vi "NNScoreImage.vi"(0 "lookup path":path, 1 "Window Av Size":i8=3, 2 "psa":dbl format="%.2f", 3 "Intercept":dbl[][](array[numeric]) format="%.2f", 4 "MidBand":dbl[][](array[numeric]) format="%.2f") -> (6 "score":dbl[][](graph), 7 "Range Params":T1={"mb max"=-10.0, "mb min"=-60.0, "slope max"=4.0, "slope min"=-8.0, "int max"=5.0, "int min"=-85.0} {"int min" format="%.2f"; "int max" format="%.2f"; "slope min" format="%.2f"; "slope max" format="%.2f"; "mb min" format="%.2f"; "mb max" format="%.2f"}, 10 "Range Params in LUT":T1={"mb max"=-20.0, "mb min"=-70.0, "slope max"=8.0, "slope min"=-8.0, "int max"=5.0, "int min"=-85.0} {"int min" format="%.2f"; "int max" format="%.2f"; "slope min" format="%.2f"; "slope max" format="%.2f"; "mb min" format="%.2f"; "mb max" format="%.2f"})   [LabVIEW 2022 SP3]
uses:
  <vilib>/Utility/file.llb/Read Delimited Spreadsheet (DBL).vi
panel:
  out "min score":sgl
  out "max score":sgl
  in  "Look Up Dimension":i32=40
  out "Look up Table":dbl[][][](array[numeric]) format="%.6f"
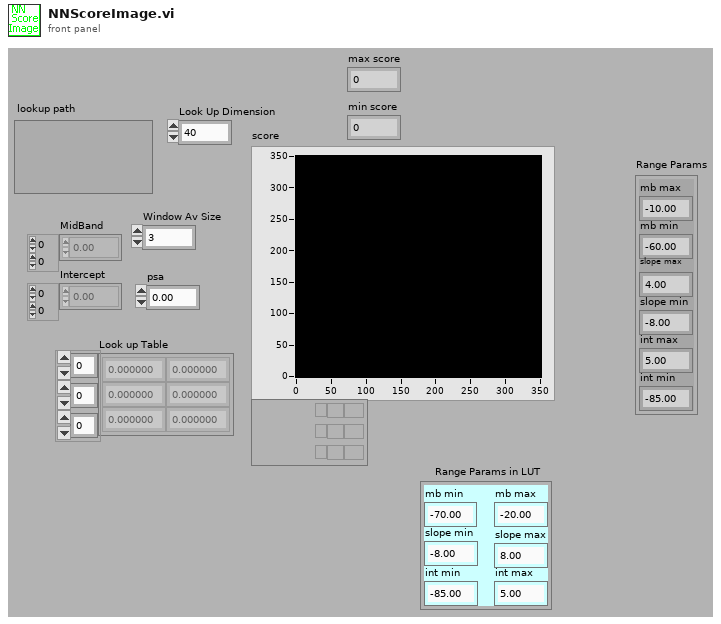
[diagram p1: front panel]
types:
  T1 = cluster{"mb max":dbl, "mb min":dbl, "slope max":dbl, "slope min":dbl, "int max":dbl, "int min":dbl}
  T2 = cluster{"[0]":dbl, "[1]":dbl, "[2]":dbl, "[3]":dbl, "[4]":dbl, "[5]":dbl, "[6]":dbl, "[7]":dbl}
  T3 = cluster{"[5]":dbl, "[4]":dbl, "[1]":dbl, "[0]":dbl, "[3]":dbl, "[2]":dbl}
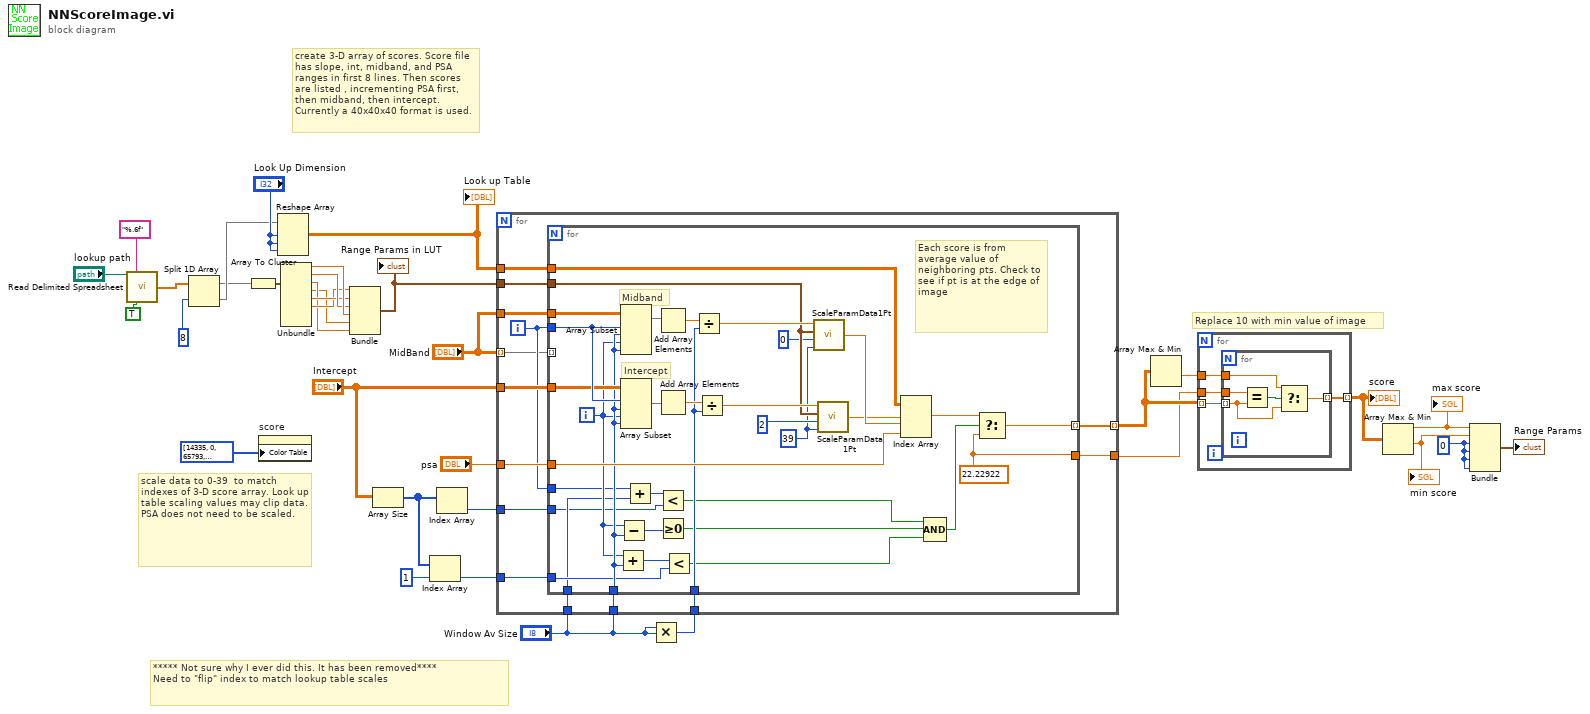
[diagram p0: block diagram]
diagram:
  w8 = 0
  # "***** Not sure why I ever did this. It has been removed****\nNeed to \"flip\" index to match lookup table scales"
  # "Replace 10 with min value of image"
  # "scale data to 0-39  to match indexes of 3-D score array. Look up table scaling values may clip data. PSA does not need to be scaled."
  # "create 3-D array of scores. Score file has slope, int, midband, and PSA ranges in first 8 lines. Then scores are listed , incrementing PSA first, then midband, then intercept.  Currently a 40x40x40 format is used."
  n1 = call-poly <vilib>:"Read Delimited Spreadsheet.vi"("file path (dialog if empty)"="lookup path", "format (%.3f)"="%.6f", "transpose? (F)"=TRUE) -> ("first row"=w7:dbl[])  [unwired: 7 in, 5 out]
  n2 = Split 1D Array(array=w7, index=8) -> (first subarray=w4:dbl[], second subarray=w5:dbl[])
  n3 = Array To Cluster(array=w4) -> (cluster=w32:T2)
  n4 = property on="score" class="IntGraph (strict)"("Color Table"=u32[] [14335, 0, 65793, 131586, 197379, 263172, 328965, 394758, 460551, 526344, 592137, 657930, 723723, 789516, 855309, 921102, 986895, 1052688, 1118481, 1184274, 1250067, 1315860, 1381653, 1447446, 1513239, 1579032, 1644825, 1710618, 1776411, 1842204, 1907997, 1973790, 2039583, 2105376, 2171169, 2236962, 2302755, 2368548, 2434341, 2500134, 2565927, 2631720, 2697513, 2763306, 2829099, 2894892, 2960685, 3026478, 3092271, 3158064, 3223857, 3289650, 3355443, 3421236, 3487029, 3552822, 3618615, 3684408, 3750201, 3815994, 3881787, 3947580, 4013373, 4079166, 4144959, 4210752, 4276545, 4342338, 4408131, 4473924, 4539717, 4605510, 4671303, 4737096, 4802889, 4868682, 4934475, 5000268, 5066061, 5131854, 5197647, 5263440, 5329233, 5395026, 5460819, 5526612, 5592405, 5658198, 5723991, 5789784, 5855577, 5921370, 5987163, 6052956, 6118749, 6184542, 6250335, 6316128, 6381921, 6447714, 6513507, 6579300, 6645093, 6710886, 6776679, 6842472, 6908265, 6974058, 7039851, 7105644, 7171437, 7237230, 7303023, 7368816, 7434609, 7500402, 7566195, 7631988, 7697781, 7763574, 7829367, 7895160, 7960953, 8026746, 8092539, 8158332, 8224125, 8289918, 8355711, 8421504, 8487297, 8553090, 8618883, 8684676, 8750469, 8816262, 8882055, 8947848, 9013641, 9079434, 9145227, 9211020, 9276813, 9342606, 9408399, 9474192, 9539985, 9605778, 9671571, 9737364, 9803157, 9868950, 9934743, 10000536, 10066329, 10132122, 10197915, 10263708, 10329501, 10395294, 10461087, 10526880, 10592673, 10658466, 10724259, 10790052, 10855845, 10921638, 10987431, 11053224, 11119017, 11184810, 11250603, 11316396, 11382189, 11447982, 11513775, 11579568, 11645361, 11711154, 11776947, 11842740, 11908533, 11974326, 12040119, 12105912, 12171705, 12237498, 12303291, 12369084, 12434877, 12500670, 12566463, 12632256, 12698049, 12763842, 12829635, 12895428, 12961221, 13027014, 13092807, 13158600, 13224393, 13290186, 13355979, 13421772, 13487565, 13553358, 13619151, 13684944, 13750737, 13816530, 13882323, 13948116, 14013909, 14079702, 14145495, 14211288, 14277081, 14342874, 14408667, 14474460, 14540253, 14606046, 14671839, 14737632, 14803425, 14869218, 14935011, 15000804, 15066597, 15132390, 15198183, 15263976, 15329769, 15395562, 15461355, 15527148, 15592941, 15658734, 15724527, 15790320, 15856113, 15921906, 15987699, 16053492, 16119285, 16185078, 16250871, 16316664, 16382457, 16448250, 16514043, 16579836, 16758546, 16711731]) -> ()  [unwired: 2 in, 2 out]
  n5 = Reshape Array(w5, "Look Up Dimension", "Look Up Dimension", "Look Up Dimension") -> (w10:dbl[][][])
  "Look up Table" <- w10
  n6 = Unbundle(w32) -> ("[0]"=w31:dbl, "[1]"=w30:dbl, "[2]"=w27:dbl, "[3]"=w26:dbl, "[4]"=w29:dbl, "[5]"=w28:dbl)  [unwired: 2 out]
  n7 = Bundle("[5]"=w28, "[4]"=w29, "[1]"=w30, "[0]"=w31, "[3]"=w26, "[2]"=w27) -> (w3:T3)  [unwired: 1 out]
  "Range Params in LUT" <- w3
  n8 = Array Size(array="Intercept") -> (size(s)=w14:i32[])
  n9 = Index Array(array=w14, index=1) -> (element=w17:i32)
  n10 = Index Array(array=w14) -> (element=w13:i32)  [unwired: 1 in]
  n11 = Multiply(x="Window Av Size", y="Window Av Size") -> (x*y=w22:i8)
  n12 = for {
    tunnel: w10 -> [w49]
    tunnel: "psa" -> [w48]
    tunnel: [w47] -> w19 mode=indexing
    tunnel: "MidBand" -> [w46]
    tunnel: "Intercept" -> [w45]
    tunnel: "Window Av Size" -> [w44]
    tunnel: w22 -> [w43]
    tunnel: [w42] -> w18
    tunnel: w17 -> [w41]
    tunnel: "Window Av Size" -> [w40]
    tunnel: w13 -> [w38]
    tunnel: "MidBand" -> [w37] mode=indexing
    tunnel: w3 -> [w36]
    i -> [w39]
    n13 = for {
      tunnel: w49 -> [w82]
      tunnel: w48 -> [w83]
      tunnel: [w71] -> w47 mode=indexing
      tunnel: w39 -> [w81]
      tunnel: w46 -> [w80]
      tunnel: w45 -> [w79]
      tunnel: w44 -> [w73]
      tunnel: w43 -> [w74]
      tunnel: [w69] -> w42
      tunnel: w41 -> [w64]
      tunnel: w40 -> [w62]
      tunnel: w39 -> [w61]
      tunnel: w38 -> [w59]
      tunnel: w37 -> [_] mode=indexing
      tunnel: w36 -> [w53]
      i -> [w68]
      w50 = 39
      w69 = 22.22922
      # "Each score is from average value of neighboring pts. Check to see if pt is at the edge of image"
      # "Intercept"
      # "Midband"
      n14 = Add(x=w68, y=w73) -> (x+y=w63:i32)
      n15 = Subtract(x=w68, y=w73) -> (x-y=w67:i32)
      n16 = Array Subset(array=w80, index (row)=w81, length (row)=w73, index (col)=w68, length (col)=w73) -> (w78:dbl[][])
      n17 = Array Subset(array=w79, index (row)=w81, length (row)=w73, index (col)=w68, length (col)=w73) -> (w77:dbl[][])
      n18 = Add(x=w61, y=w62) -> (x+y=w60:i32)
      n19 = Add Array Elements(numeric array=w78) -> (sum=w75:dbl)
      n20 = Add Array Elements(numeric array=w77) -> (sum=w76:dbl)
      n21 = Less?(x=w60, y=w59) -> (x < y?=w58:bool)
      n22 = Greater Or Equal To 0?(x=w67) -> (x >= 0?=w66:bool)
      n23 = Less?(x=w63, y=w64) -> (x < y?=w65:bool)
      n24 = Divide(x=w75, y=w74) -> (x/y=w57:dbl)
      n25 = Divide(x=w76, y=w74) -> (x/y=w54:dbl)
      n26 = call "ScaleParamData1Pt.vi"("max scale value"=w50, "parameter"=0, "Range Params"=w53, "raw image data in"=w57) -> ("scaled output"=w56:dbl)
      n27 = call "ScaleParamData1Pt.vi"("max scale value"=w50, "parameter"=2, "Range Params"=w53, "raw image data in"=w54) -> ("scaled output"=w55:dbl)
      n28 = Index Array(array=w82, index (dim 0)=w55, index (dim 1)=w56, index (dim 2)=w83) -> (element=w72:dbl)
      n29 = Compound Arithmetic op=AND(w58, w66, w65) -> (w70:bool)
      n30 = Select(t=w72, s=w70, f=w69) -> (s? t:f=w71:dbl)
    }
  }
  n31 = Array Max & Min(array=w19) -> (min value=w20:dbl)  [unwired: 3 out]
  n32 = for {
    tunnel: [w87] -> w9 mode=indexing
    tunnel: w19 -> [w86] mode=indexing
    tunnel: w18 -> [w85]
    tunnel: w20 -> [w84]
    n33 = for {
      tunnel: [w91] -> w87 mode=indexing
      tunnel: w86 -> [w88] mode=indexing
      tunnel: w85 -> [w90]
      tunnel: w84 -> [w89]
      n34 = Equal?(x=w90, y=w88) -> (x = y?=w92:bool)
      n35 = Select(t=w89, s=w92, f=w88) -> (s? t:f=w91:dbl)
    }
  }
  "score" <- w9
  n36 = Array Max & Min(array=w9) -> (max value=w12:dbl, min value=w11:dbl)  [unwired: 2 out]
  "max score" <- w12
  "min score" <- w11
  n37 = Bundle(w12, w11, w8, w8, w8, w8) -> (→"Range Params":cluster{dbl, dbl, i32, i32, i32, i32})  [unwired: 1 out]
